vi "Anritsu VNA Read Calibration Status.vi"(7 "Anritsu VNA":T6, 8 "error in (no error)":errorcluster, 10 "Parameters to Measure":T2[](array[typedef]) {"Channel" min=1 max=99 step=1; "Parameter"."Stimulus Port" min=1 step=1; "Parameter"."Response Port" min=1 step=1}, 11 "VISA Resource Name":refnum<visa-resource-name>) -> (0 "error out":errorcluster {"code" format="%.0x"}, 1 "Parameters to Measure":T2[](array[typedef]) {"Channel" min=1 max=99 step=1; "Parameter"."Stimulus Port" min=1 step=1; "Parameter"."Response Port" min=1 step=1}, 2 "Calibration Type by Parameter":T1[](array[typedef]), 3 "dup VISA Resource Name":refnum<visa-resource-name>)   [LabVIEW 2011]
doc: "This VI for the HP 8753B is used to read the calibration type.\n\n0 response\n1 response and isolation\n2 S11 1-port\n3 S22 1-port\n4 full 2-port\n5 one path 2-port\n6 no cal detected"
uses:
  TypeDefs/Anritsu VNA Instrument Info.ctl
  tests/S Parameter/TypeDefs/SP Parameter to Measure.ctl
  tests/S Parameter/TypeDefs/SP Parameter.ctl
  tests/S Parameter/TypeDefs/SP Calibration State.ctl
  tests/S Parameter/TypeDefs/SP Measurement Format.ctl
  TypeDefs/Anritsu VNA Calibration State.ctl
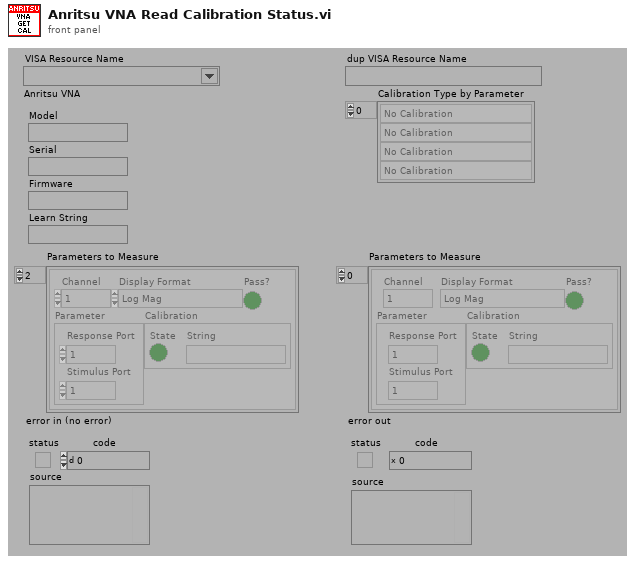
[diagram p1: front panel]
types:
  T1 = typedef "Anritsu VNA Calibration State.ctl" = enum32{"No Calibration", "12 Term (2-Port)", "8 Term FWD", "8 Term REV", "Transmission FWD", "Transmission REV", "Transmission FWD & REV", "Reflection FWD", "Reflection REV", "Reflection FWD & REV", "24 Term (3-Port)", "40 Term (4-Port)", "Full 1-Port (Port 1)", "Full 1-Port (Port 2)", "Full 1-Port (Port 1 & 2)", "Full 2-Port", "One Path 2-Port FWD", "One Path 2-Port REV"}
  T2 = typedef "SP Parameter to Measure.ctl" = cluster{"Channel":i8, "Parameter":T3, "Calibration":T4, "Display Format":T5, "Pass?":bool}
  T3 = typedef "SP Parameter.ctl" = cluster{"Stimulus Port":i8, "Response Port":i8}
  T4 = typedef "SP Calibration State.ctl" = cluster{"State":bool, "String":string}
  T5 = typedef "SP Measurement Format.ctl" = enum32{"Log Mag", "Phase", "Delay", "Smith (R+jX)", "Polar (Re/Im)", "Linear Mag", "SWR", "Real", "Imaginary", "Smith (Lin/Phase)", "Smith (Log/Phase)", "Smith (Real/Imag)", "Smith (G+jB)", "Polar (Lin/Phase)", "Polar (Log/Phase)", "Expanded Phase", "Positive Phase", "Inverted Smith", "Unwrapped Phase", "Power Out", "Power In", "Linear Mag/Phase", "Log Mag/Phase", "Real/Imaginary"}
  T6 = typedef "Anritsu VNA Instrument Info.ctl" = cluster{"Model":string, "Serial":string, "Firmware":string, "Learn String":string}
  T7 = typedef "Anritsu VNA Model.ctl" = enum16{"Not Supported", "37XXXX", "MS20XXX", "MS462XX", "MS464XX"}
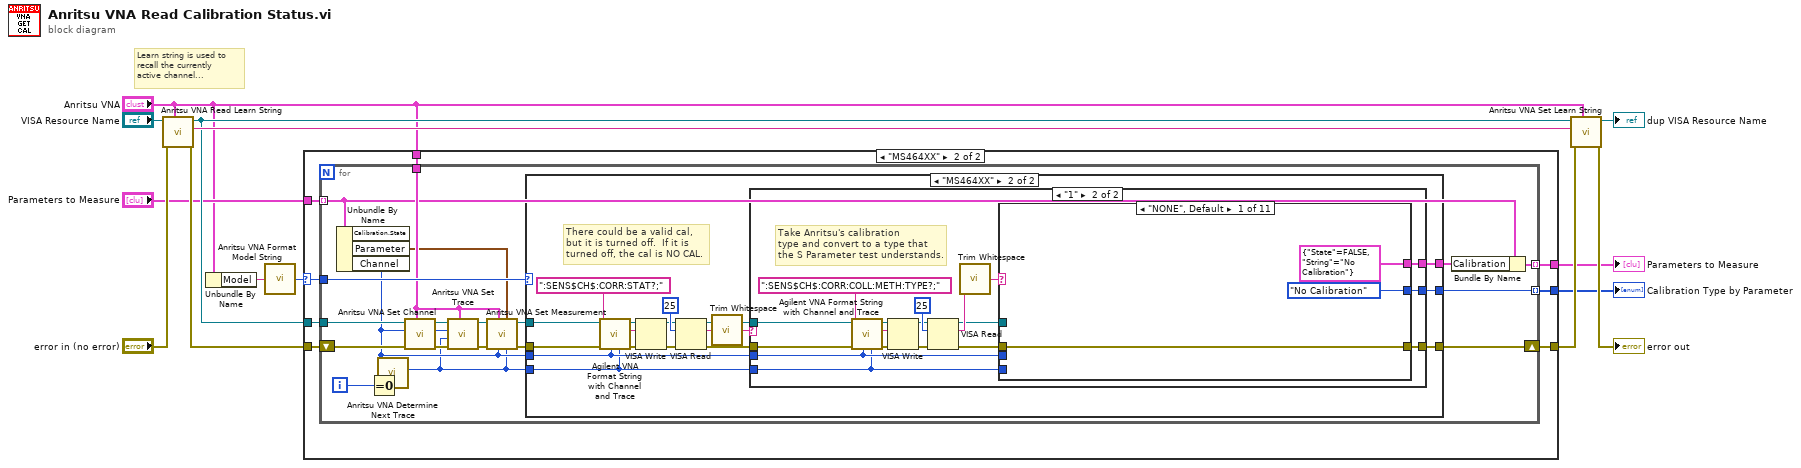
[diagram p0: block diagram]
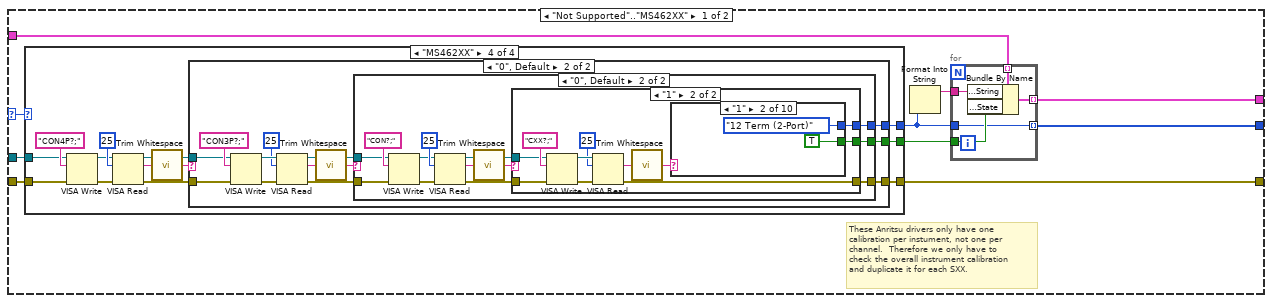
[diagram p2: hidden frame]
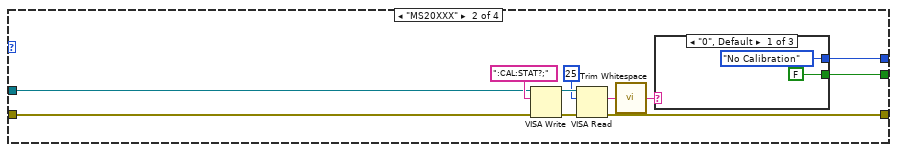
[diagram p4: hidden frame]
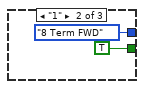
[diagram p5: hidden frame]
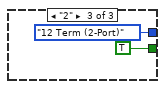
[diagram p6: hidden frame]
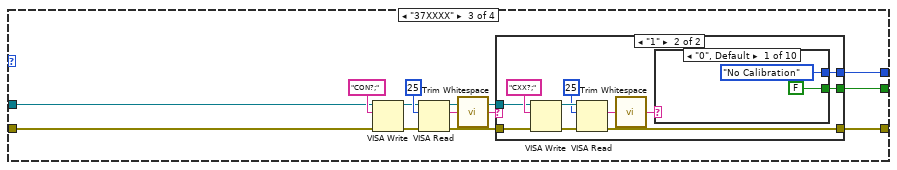
[diagram p7: hidden frame]
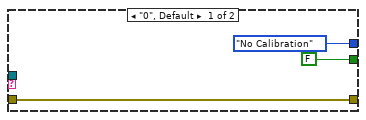
[diagram p8: hidden frame]
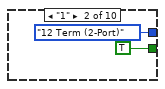
[diagram p9: hidden frame]
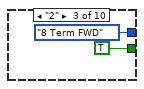
[diagram p10: hidden frame]
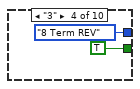
[diagram p11: hidden frame]
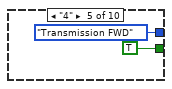
[diagram p12: hidden frame]
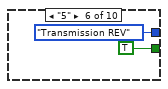
[diagram p13: hidden frame]
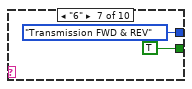
[diagram p14: hidden frame]
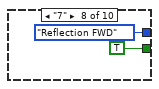
[diagram p15: hidden frame]
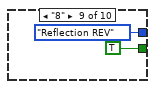
[diagram p16: hidden frame]
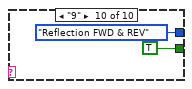
[diagram p17: hidden frame]
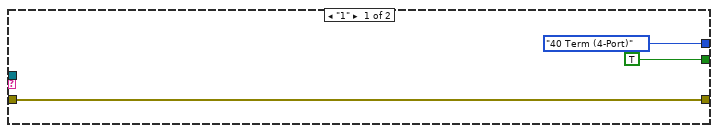
[diagram p18: hidden frame]
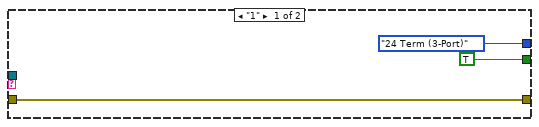
[diagram p19: hidden frame]
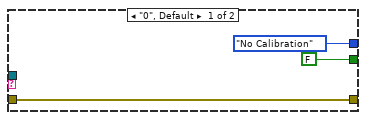
[diagram p20: hidden frame]
diagram:
  # "Learn string is used to\nrecall the currently \nactive channel..."
  n1 = call "Anritsu VNA Read Learn String.vi"("Anritsu VNA"="Anritsu VNA", "error in (no error)"="error in (no error)", "VISA Resource Name"="VISA Resource Name") -> ("error out"=w4:errorcluster, "Learn String"=w12:string, "dup VISA Resource Name"=w5:refnum<visa-resource-name>)  [unwired: 6 out]
  n2 = Unbundle By Name("Anritsu VNA") -> ("Model"=w8:string)
  n3 = call "Anritsu VNA Format Model String.vi"("Model"=w8) -> ("Model"=w1:T7)
  n4 = case shown="\"MS464XX\"" w1 {
    selector: w1 -> [w17 w176]
    tunnel: [w24 w181] -> w11
    tunnel: [w20 w175] -> w7
    tunnel: [w19 w174] -> w6
    tunnel: w5 -> [w16 w180]
    tunnel: w4 -> [w15 w179]
    tunnel: "Parameters to Measure" -> [w18 w178]
    tunnel: "Anritsu VNA" -> [_ w177]
    frame "Not Supported".."MS462XX" {
      # "These Anritsu drivers only have one\ncalibration per instument, not one per\nchannel.  Therefore we only have to\ncheck the overall instrument calibration\nand duplicate it for each SXX."
      n5 = case shown="\"MS462XX\"" w17 {
        tunnel: w15 -> [w25 w31 w46 w91]
        tunnel: w16 -> [_ w32 w47 w92]
        tunnel: [w25 w29 w45 w101] -> w24
        tunnel: [_ w30 w43 w102] -> w21
        tunnel: [_ w28 w44 w100] -> w22
        frame "Not Supported", "MS464XX" {
        }
        frame "MS20XXX" {
          n6 = VISA Write(VISA resource name=w32, write buffer=":CAL:STAT?;", error in (no error)=w31) -> (VISA resource name out=w35:refnum<visa-resource-name>, error out=w33:errorcluster)  [unwired: 1 out]
          n7 = VISA Read(VISA resource name=w35, byte count=u32 25, error in (no error)=w33) -> (read buffer=w27:string, error out=w29:errorcluster)  [unwired: 2 out]
          n8 = call <vilib>:"Trim Whitespace.vi"("string"=w27) -> ("trimmed string"=w26:string)  [unwired: 1 in]
          n9 = case shown="\"0\", Default" w26 {
            tunnel: [Anritsu_VNA_Calibration_State."No Calibration" ("VNA Calibration to Perform (not calibrated)") Anritsu_VNA_Calibration_State."8 Term FWD" ("VNA Calibration to Perform (not calibrated)") Anritsu_VNA_Calibration_State."12 Term (2-Port)" ("VNA Calibration to Perform (not calibrated)")] -> w30
            tunnel: [FALSE TRUE TRUE] -> w28
            frame "0", Default {
            }
            frame "1" {
            }
            frame "2" {
            }
          }
        }
        frame "37XXXX" {
          n10 = VISA Write(VISA resource name=w47, write buffer="CON?;", error in (no error)=w46) -> (VISA resource name out=w52:refnum<visa-resource-name>, error out=w54:errorcluster)  [unwired: 1 out]
          n11 = VISA Read(VISA resource name=w52, byte count=u32 25, error in (no error)=w54) -> (VISA resource name out=w48:refnum<visa-resource-name>, read buffer=w55:string, error out=w49:errorcluster)  [unwired: 1 out]
          n12 = call <vilib>:"Trim Whitespace.vi"("string"=w55) -> ("trimmed string"=w50:string)  [unwired: 1 in]
          n13 = case shown="\"1\"" w50 {
            tunnel: w48 -> [_ w65]
            tunnel: w49 -> [w56 w64]
            tunnel: [Anritsu_VNA_Calibration_State."No Calibration" ("VNA Calibration to Perform (not calibrated)") w60] -> w43
            tunnel: [w56 w63] -> w45
            tunnel: [FALSE w61] -> w44
            frame "0", Default {
            }
            frame "1" {
              n14 = VISA Write(VISA resource name=w65, write buffer="CXX?;", error in (no error)=w64) -> (VISA resource name out=w68:refnum<visa-resource-name>, error out=w66:errorcluster)  [unwired: 1 out]
              n15 = VISA Read(VISA resource name=w68, byte count=u32 25, error in (no error)=w66) -> (read buffer=w62:string, error out=w63:errorcluster)  [unwired: 2 out]
              n16 = call <vilib>:"Trim Whitespace.vi"("string"=w62) -> ("trimmed string"=w59:string)  [unwired: 1 in]
              n17 = case shown="\"0\", Default" w59 {
                tunnel: [Anritsu_VNA_Calibration_State."No Calibration" ("VNA Calibration to Perform (not calibrated)") Anritsu_VNA_Calibration_State."12 Term (2-Port)" ("VNA Calibration to Perform (not calibrated)") Anritsu_VNA_Calibration_State."8 Term FWD" ("VNA Calibration to Perform (not calibrated)") Anritsu_VNA_Calibration_State."8 Term REV" ("VNA Calibration to Perform (not calibrated)") Anritsu_VNA_Calibration_State."Transmission FWD" ("VNA Calibration to Perform (not calibrated)") Anritsu_VNA_Calibration_State."Transmission REV" ("VNA Calibration to Perform (not calibrated)") Anritsu_VNA_Calibration_State."Transmission FWD & REV" ("VNA Calibration to Perform (not calibrated)") Anritsu_VNA_Calibration_State."Reflection FWD" ("VNA Calibration to Perform (not calibrated)") Anritsu_VNA_Calibration_State."Reflection REV" ("VNA Calibration to Perform (not calibrated)") Anritsu_VNA_Calibration_State."Reflection FWD & REV" ("VNA Calibration to Perform (not calibrated)")] -> w60
                tunnel: [FALSE TRUE TRUE TRUE TRUE TRUE TRUE TRUE TRUE TRUE] -> w61
                frame "0", Default {
                }
                frame "1" {
                }
                frame "2" {
                }
                frame "3" {
                }
                frame "4" {
                }
                frame "5" {
                }
                frame "6" {
                }
                frame "7" {
                }
                frame "8" {
                }
                frame "9" {
                }
              }
            }
          }
        }
        frame "MS462XX" {
          n18 = VISA Write(VISA resource name=w92, write buffer="CON4P?;", error in (no error)=w91) -> (VISA resource name out=w96:refnum<visa-resource-name>, error out=w98:errorcluster)  [unwired: 1 out]
          n19 = VISA Read(VISA resource name=w96, byte count=u32 25, error in (no error)=w98) -> (VISA resource name out=w93:refnum<visa-resource-name>, read buffer=w99:string, error out=w90:errorcluster)  [unwired: 1 out]
          n20 = call <vilib>:"Trim Whitespace.vi"("string"=w99) -> ("trimmed string"=w94:string)  [unwired: 1 in]
          n21 = case shown="\"0\", Default" w94 {
            tunnel: w90 -> [w105 w107]
            tunnel: [Anritsu_VNA_Calibration_State."40 Term (4-Port)" ("VNA Calibration to Perform (not calibrated)") w118] -> w102
            tunnel: [w105 w117] -> w101
            tunnel: [TRUE w116] -> w100
            tunnel: w93 -> [_ w108]
            frame "1" {
            }
            frame "0", Default {
              n22 = VISA Write(VISA resource name=w108, write buffer="CON3P?;", error in (no error)=w107) -> (VISA resource name out=w114:refnum<visa-resource-name>, error out=w112:errorcluster)  [unwired: 1 out]
              n23 = VISA Read(VISA resource name=w114, byte count=u32 25, error in (no error)=w112) -> (VISA resource name out=w109:refnum<visa-resource-name>, read buffer=w111:string, error out=w106:errorcluster)  [unwired: 1 out]
              n24 = call <vilib>:"Trim Whitespace.vi"("string"=w111) -> ("trimmed string"=w110:string)  [unwired: 1 in]
              n25 = case shown="\"0\", Default" w110 {
                tunnel: w109 -> [_ w125]
                tunnel: w106 -> [w121 w124]
                tunnel: [Anritsu_VNA_Calibration_State."24 Term (3-Port)" ("VNA Calibration to Perform (not calibrated)") w134] -> w118
                tunnel: [w121 w133] -> w117
                tunnel: [TRUE w132] -> w116
                frame "1" {
                }
                frame "0", Default {
                  n26 = VISA Write(VISA resource name=w125, write buffer="CON?;", error in (no error)=w124) -> (VISA resource name out=w128:refnum<visa-resource-name>, error out=w130:errorcluster)  [unwired: 1 out]
                  n27 = VISA Read(VISA resource name=w128, byte count=u32 25, error in (no error)=w130) -> (VISA resource name out=w122:refnum<visa-resource-name>, read buffer=w131:string, error out=w123:errorcluster)  [unwired: 1 out]
                  n28 = call <vilib>:"Trim Whitespace.vi"("string"=w131) -> ("trimmed string"=w126:string)  [unwired: 1 in]
                  n29 = case shown="\"1\"" w126 {
                    tunnel: w122 -> [_ w144]
                    tunnel: w123 -> [w135 w143]
                    tunnel: [Anritsu_VNA_Calibration_State."No Calibration" ("VNA Calibration to Perform (not calibrated)") w142] -> w134
                    tunnel: [w135 w141] -> w133
                    tunnel: [FALSE w140] -> w132
                    frame "0", Default {
                    }
                    frame "1" {
                      n30 = VISA Write(VISA resource name=w144, write buffer="CXX?;", error in (no error)=w143) -> (VISA resource name out=w147:refnum<visa-resource-name>, error out=w145:errorcluster)  [unwired: 1 out]
                      n31 = VISA Read(VISA resource name=w147, byte count=u32 25, error in (no error)=w145) -> (read buffer=w139:string, error out=w141:errorcluster)  [unwired: 2 out]
                      n32 = call <vilib>:"Trim Whitespace.vi"("string"=w139) -> ("trimmed string"=w138:string)  [unwired: 1 in]
                      n33 = case shown="\"1\"" w138 {
                        tunnel: [Anritsu_VNA_Calibration_State."No Calibration" ("VNA Calibration to Perform (not calibrated)") Anritsu_VNA_Calibration_State."12 Term (2-Port)" ("VNA Calibration to Perform (not calibrated)") Anritsu_VNA_Calibration_State."8 Term FWD" ("VNA Calibration to Perform (not calibrated)") Anritsu_VNA_Calibration_State."8 Term REV" ("VNA Calibration to Perform (not calibrated)") Anritsu_VNA_Calibration_State."Transmission FWD" ("VNA Calibration to Perform (not calibrated)") Anritsu_VNA_Calibration_State."Transmission REV" ("VNA Calibration to Perform (not calibrated)") Anritsu_VNA_Calibration_State."Transmission FWD & REV" ("VNA Calibration to Perform (not calibrated)") Anritsu_VNA_Calibration_State."Reflection FWD" ("VNA Calibration to Perform (not calibrated)") Anritsu_VNA_Calibration_State."Reflection REV" ("VNA Calibration to Perform (not calibrated)") Anritsu_VNA_Calibration_State."Reflection FWD & REV" ("VNA Calibration to Perform (not calibrated)")] -> w142
                        tunnel: [FALSE TRUE TRUE TRUE TRUE TRUE TRUE TRUE TRUE TRUE] -> w140
                        frame "0", Default {
                        }
                        frame "1" {
                        }
                        frame "2" {
                        }
                        frame "3" {
                        }
                        frame "4" {
                        }
                        frame "5" {
                        }
                        frame "6" {
                        }
                        frame "7" {
                        }
                        frame "8" {
                        }
                        frame "9" {
                        }
                      }
                    }
                  }
                }
              }
            }
          }
        }
      }
      n34 = Format Into String(w21) -> (resulting string=w23:string)  [unwired: 3 in, 1 out]
      n35 = for {
        tunnel: w18 -> [w173] mode=indexing
        tunnel: w23 -> [w172]
        tunnel: w22 -> [w171]
        tunnel: w21 -> [w170]
        tunnel: [w170] -> w20 mode=indexing
        tunnel: [w169] -> w19 mode=indexing
        n36 = Bundle By Name(cluster=w173, "Calibration.String"=w172, "Calibration.State"=w171) -> (w169:T2)
      }
    }
    frame "MS464XX" {
      n37 = for {
        tunnel: w176 -> [w200]
        tunnel: [w199] -> w175 mode=indexing
        tunnel: w180 -> [w195]
        shift-right: [w201] -> w181
        shift-left: w179 -> [w196]
        tunnel: w178 -> [w183] mode=indexing
        tunnel: w177 -> [w188]
        tunnel: [w182] -> w174 mode=indexing
        i -> [w197]
        n38 = Unbundle By Name(w183) -> ("Parameter"=w187:T3, "Channel"=w186:i8)  [unwired: 1 out]
        n39 = Equal To 0?(x=w197) -> (x = 0?=w198:bool)
        n40 = call "Anritsu VNA Determine Next Trace.vi"("Reset?"=w198, "Channel"=w186) -> ("Next Trace"=w185:i8)  [unwired: 9 out]
        n41 = call "Anritsu VNA Set Channel.vi"("Anritsu VNA"=w188, "error in (no error)"=w196, "Channel"=w186, "VISA Resource Name"=w195) -> ("error out"=w191:errorcluster, "dup VISA Resource Name"=w192:refnum<visa-resource-name>)  [unwired: 6 out]
        n42 = call "Anritsu VNA Set Trace.vi"("Anritsu VNA"=w188, "error in (no error)"=w191, "Trace"=w185, "Channel"=w186, "VISA Resource Name"=w192) -> ("error out"=w190:errorcluster, "dup VISA Resource Name"=w189:refnum<visa-resource-name>)  [unwired: 5 out]
        n43 = call "Anritsu VNA Set Measurement.vi"("Trace"=w185, "Parameter"=w187, "Channel"=w186, "Anritsu VNA"=w188, "error in (no error)"=w190, "VISA Resource Name"=w189) -> ("error out"=w193:errorcluster, "dup VISA Resource Name"=w194:refnum<visa-resource-name>)  [unwired: 4 out]
        n44 = case shown="\"MS464XX\"" w200 {
          tunnel: w193 -> [w202 w209]
          tunnel: w194 -> [_ w208]
          tunnel: [w202 w205] -> w201
          tunnel: [_ w204] -> w199
          tunnel: w186 -> [_ w207]
          tunnel: w185 -> [_ w206]
          tunnel: [_ w203] -> w184
          frame "Not Supported".."MS462XX" {
          }
          frame "MS464XX" {
            # "There could be a valid cal,\nbut it is turned off.  If it is\nturned off, the cal is NO CAL."
            n45 = call "Agilent VNA Format String with Channel and Trace.vi"("Trace"=w206, "Channel"=w207, "String"=":SENS$CH$:CORR:STAT?;") -> ("String Out"=w218:string)  [unwired: 6 out]
            n46 = VISA Write(VISA resource name=w208, write buffer=w218, error in (no error)=w209) -> (VISA resource name out=w213:refnum<visa-resource-name>, error out=w216:errorcluster)  [unwired: 1 out]
            n47 = VISA Read(VISA resource name=w213, byte count=u32 25, error in (no error)=w216) -> (VISA resource name out=w214:refnum<visa-resource-name>, read buffer=w211:string, error out=w215:errorcluster)  [unwired: 1 out]
            n48 = call <vilib>:"Trim Whitespace.vi"("string"=w211) -> ("trimmed string"=w210:string)  [unwired: 1 in]
            n49 = case shown="\"1\"" w210 {
              tunnel: [Anritsu_VNA_Calibration_State."No Calibration" ("S Parameter Test Cal Type") w237] -> w204
              tunnel: w215 -> [w219 w231]
              tunnel: w214 -> [_ w230]
              tunnel: [w219 w226] -> w205
              tunnel: [T4 {"State"=FALSE, "String"="No Calibration"} w225] -> w203
              tunnel: w207 -> [_ w224]
              tunnel: w206 -> [_ w223]
              frame "0", Default {
              }
              frame "1" {
                # "Take Anritsu's calibration\ntype and convert to a type that\nthe S Parameter test understands."
                n50 = call "Agilent VNA Format String with Channel and Trace.vi"("Trace"=w223, "Channel"=w224, "String"=":SENS$CH$:CORR:COLL:METH:TYPE?;") -> ("String Out"=w234:string)  [unwired: 6 out]
                n51 = VISA Write(VISA resource name=w230, write buffer=w234, error in (no error)=w231) -> (VISA resource name out=w235:refnum<visa-resource-name>, error out=w229:errorcluster)  [unwired: 1 out]
                n52 = VISA Read(VISA resource name=w235, byte count=u32 25, error in (no error)=w229) -> (VISA resource name out=w227:refnum<visa-resource-name>, read buffer=w232:string, error out=w228:errorcluster)  [unwired: 1 out]
                n53 = call <vilib>:"Trim Whitespace.vi"("string"=w232) -> ("trimmed string"=w222:string)  [unwired: 1 in]
                n54 = case shown="\"NONE\", Default" w222 {
                  tunnel: [Anritsu_VNA_Calibration_State."No Calibration" ("S Parameter Test Cal Type") Anritsu_VNA_Calibration_State."Reflection FWD" ("S Parameter Test Cal Type") Anritsu_VNA_Calibration_State."Reflection FWD & REV" ("S Parameter Test Cal Type") w258 Anritsu_VNA_Calibration_State."Full 2-Port" ("S Parameter Test Cal Type") Anritsu_VNA_Calibration_State."Full 1-Port (Port 1 & 2)" ("S Parameter Test Cal Type") Anritsu_VNA_Calibration_State."Transmission FWD" ("S Parameter Test Cal Type") Anritsu_VNA_Calibration_State."Transmission REV" ("S Parameter Test Cal Type") Anritsu_VNA_Calibration_State."Transmission FWD & REV" ("S Parameter Test Cal Type") Anritsu_VNA_Calibration_State."One Path 2-Port FWD" ("S Parameter Test Cal Type") Anritsu_VNA_Calibration_State."One Path 2-Port REV" ("S Parameter Test Cal Type")] -> w237
                  tunnel: w228 -> [w239 w242 w245 w251 w264 w267 w270 w273 w276 w279 w282]
                  tunnel: w224 -> [_ _ _ _ _ _ _ _ _ _ _]
                  tunnel: [w239 w242 w245 w249 w264 w267 w270 w273 w276 w279 w282] -> w226
                  tunnel: w227 -> [_ _ _ w248 _ _ _ _ _ _ _]
                  tunnel: [T4 {"State"=FALSE, "String"="No Calibration"} T4 {"State"=TRUE, "String"="Reflection FWD"} T4 {"State"=TRUE, "String"="Reflection FWD & REV"} w257 T4 {"State"=TRUE, "String"="Full 2-Port"} T4 {"State"=TRUE, "String"="Full 1-Port (Port 1 & 2)"} T4 {"State"=TRUE, "String"="Transmission FWD"} T4 {"State"=TRUE, "String"="Transmission REV"} T4 {"State"=TRUE, "String"="Transmission FWD & REV"} T4 {"State"=TRUE, "String"="One Path 2-Port FWD"} T4 {"State"=TRUE, "String"="One Path 2-Port REV"}] -> w225
                  tunnel: w223 -> [_ _ _ _ _ _ _ _ _ _ _]
                  frame "NONE", Default {
                  }
                  frame "RESP1" {
                  }
                  frame "RESP1,RESP1" {
                  }
                  frame "FULL1" {
                    n55 = call "Agilent VNA Format String with Channel and Trace.vi"("String"=":SENS$CH$:CORR:COLL:METH:PORT?;") -> ("String Out"=w254:string)  [unwired: 2 in, 6 out]
                    n56 = VISA Write(VISA resource name=w248, write buffer=w254, error in (no error)=w251) -> (VISA resource name out=w253:refnum<visa-resource-name>, error out=w250:errorcluster)  [unwired: 1 out]
                    n57 = VISA Read(VISA resource name=w253, byte count=u32 25, error in (no error)=w250) -> (read buffer=w256:string, error out=w249:errorcluster)  [unwired: 2 out]
                    n58 = call <vilib>:"Trim Whitespace.vi"("string"=w256) -> ("trimmed string"=w247:string)  [unwired: 1 in]
                    n59 = case shown="\"PORT1\", Default" w247 {
                      tunnel: [Anritsu_VNA_Calibration_State."Full 1-Port (Port 1)" ("S Parameter Test Cal Type") Anritsu_VNA_Calibration_State."Full 1-Port (Port 2)" ("S Parameter Test Cal Type")] -> w258
                      tunnel: [T4 {"State"=TRUE, "String"="Full 1-Port (Port 1)"} T4 {"State"=TRUE, "String"="Full 1-Port (Port 2)"}] -> w257
                      frame "PORT1", Default {
                      }
                      frame "PORT2" {
                      }
                    }
                  }
                  frame "FULL2" {
                  }
                  frame "FULL1,FULL1" {
                  }
                  frame "TFRF" {
                  }
                  frame "TFRR" {
                  }
                  frame "TFRB" {
                  }
                  frame "1P2PF" {
                  }
                  frame "1P2PR" {
                  }
                }
              }
            }
          }
        }
        n60 = Bundle By Name(cluster=w183, "Calibration"=w184) -> (w182:T2)
      }
    }
  }
  "Parameters to Measure" <- w6
  "Calibration Type by Parameter" <- w7
  n61 = call "Anritsu VNA Set Learn String.vi"("Anritsu VNA"="Anritsu VNA", "error in (no error)"=w11, "Learn String"=w12, "VISA Resource Name"=w5) -> ("error out"=→"error out":errorcluster, "dup VISA Resource Name"=→"dup VISA Resource Name":refnum<visa-resource-name>)  [unwired: 6 out]
